vi "Draw.vi"(11 "DataIn":T1) -> (3 "DataOut":T1)   [LabVIEW 2017]
doc: "SubVI criada para mostrar um popup para o usuário indicando que o jogo acabou em empate."
uses:
  controls/DataIn.ctl
  controls/Tabuleiro.ctl
  controls/GameOption.ctl
  controls/Table.ctl
panel:
  in  "Sair":bool
  in  "Jogar Novamente":bool
  # "Empate"
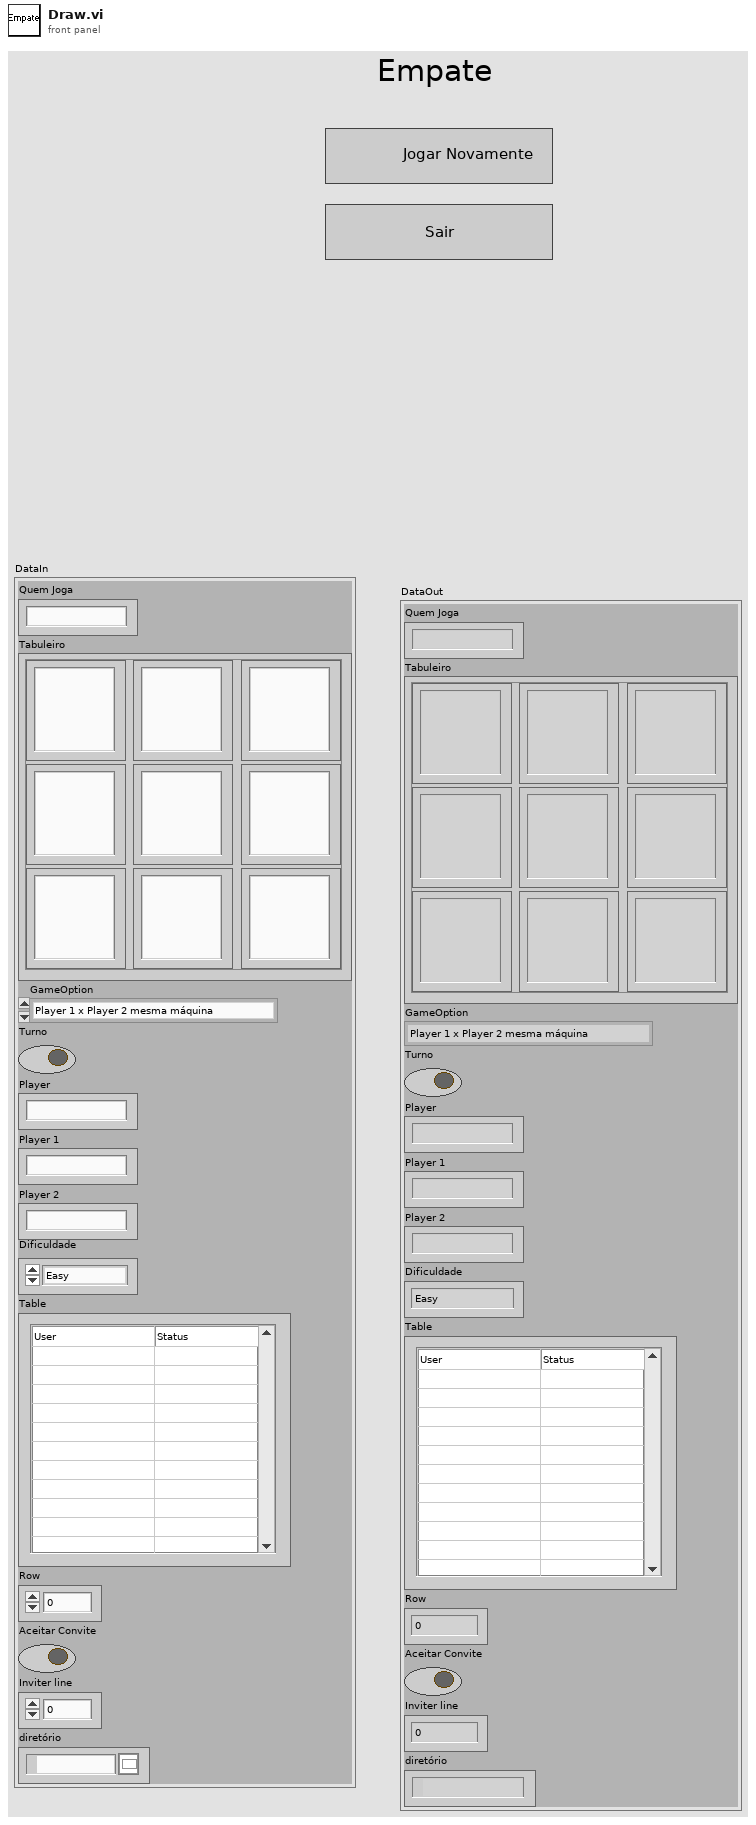
[diagram p1: front panel]
types:
  T1 = typedef "DataIn.ctl" = cluster{"Quem Joga":string, "Tabuleiro":T2, "GameOption":T3, "Turno":bool, "Player":string, "Player 1":string, "Player 2":string, "Dificuldade":enum16{"Easy", "Medium", "Hard"}, "Table":T4, "Row":u32, "Aceitar Convite":bool, "Inviter line":u32, "diretório":path}
  T2 = typedef "Tabuleiro.ctl" = cluster{"(0,0)":string, "(1,0)":string, "(0,1)":string, "(1,1)":string, "(2,0)":string, "(1,2)":string, "(2,2)":string, "(0,2)":string, "(2,1) ":string}
  T3 = typedef "GameOption.ctl" = enum16{"Player 1 x Player 2 mesma máquina", "Player 1 x Player 2 pela rede", "Player 1 x Computador", "Wait for Event", "Initialize", "Stop"}
  T4 = typedef "Table.ctl" = string[][]
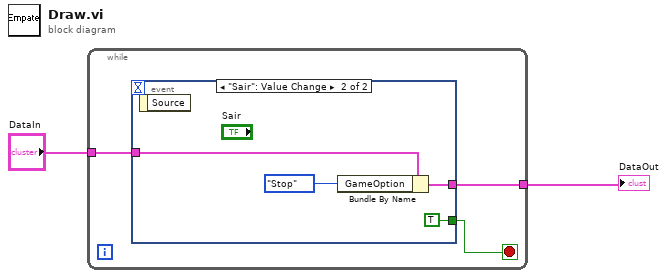
[diagram p0: block diagram]
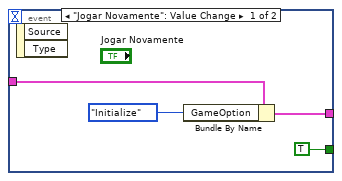
[diagram p2: hidden frame]
diagram:
  n1 = while {
    tunnel: "DataIn" -> [w5]
    tunnel: [w4] -> w1
    stop <- w3 stop-if-true
    n2 = event shown="[1] \"Sair\": Value Change" {
      selector: _ -> [_ _]
      dyn-events: _ -> [_ _]
      timeout: _ -> [_ _]
      tunnel: [w7 w13] -> w4
      tunnel: w5 -> [w8 w12]
      tunnel: [TRUE TRUE] -> w3
      event "Jogar Novamente": Value Change {
        n3 = event-data() -> ()  [unwired: 1 in, 2 out]
        n4 = Bundle By Name(cluster=w8, "GameOption"=GameOption."Initialize") -> (w7:T1)
      }
      event "Sair": Value Change {
        n5 = event-data() -> ()  [unwired: 1 in, 1 out]
        n6 = Bundle By Name(cluster=w12, "GameOption"=GameOption."Stop") -> (w13:T1)
      }
    }
  }
  "DataOut" <- w1
